vi "EditorThumbnail addNewData.vi"(7 "limit":T1={"plotIdx"=-1, "Minimum"=-inf, "Maximum"=inf}, 8 "error in (no error)":errorcluster, 11 "EditorThumbnail in":refnum<class "EditorThumbnail.lvclass">) -> (0 "error out":errorcluster, 3 "EditorThumbnail out":refnum<class "EditorThumbnail.lvclass">)   [LabVIEW 2018, in "EditorThumbnail.lvclass"]
uses:
  EditorThumbnail.lvclass
  EditorThumbnail.lvclass/EditorThumbnail.ctl
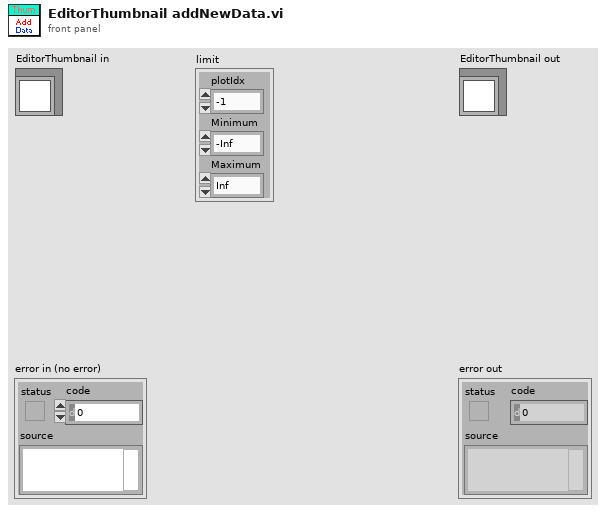
[diagram p1: front panel]
types:
  T1 = cluster{"plotIdx":i32, "Minimum":dbl, "Maximum":dbl}
  T2 = cluster{"index":u32, "data":cluster{"xdata":dbl[], "ydata":sgl[]}[], "peak":dbl[], "picture":picture}[]
  T3 = cluster{"index":u32, "data":cluster{"xdata":dbl[], "ydata":sgl[]}[], "peak":dbl[], "picture":picture}
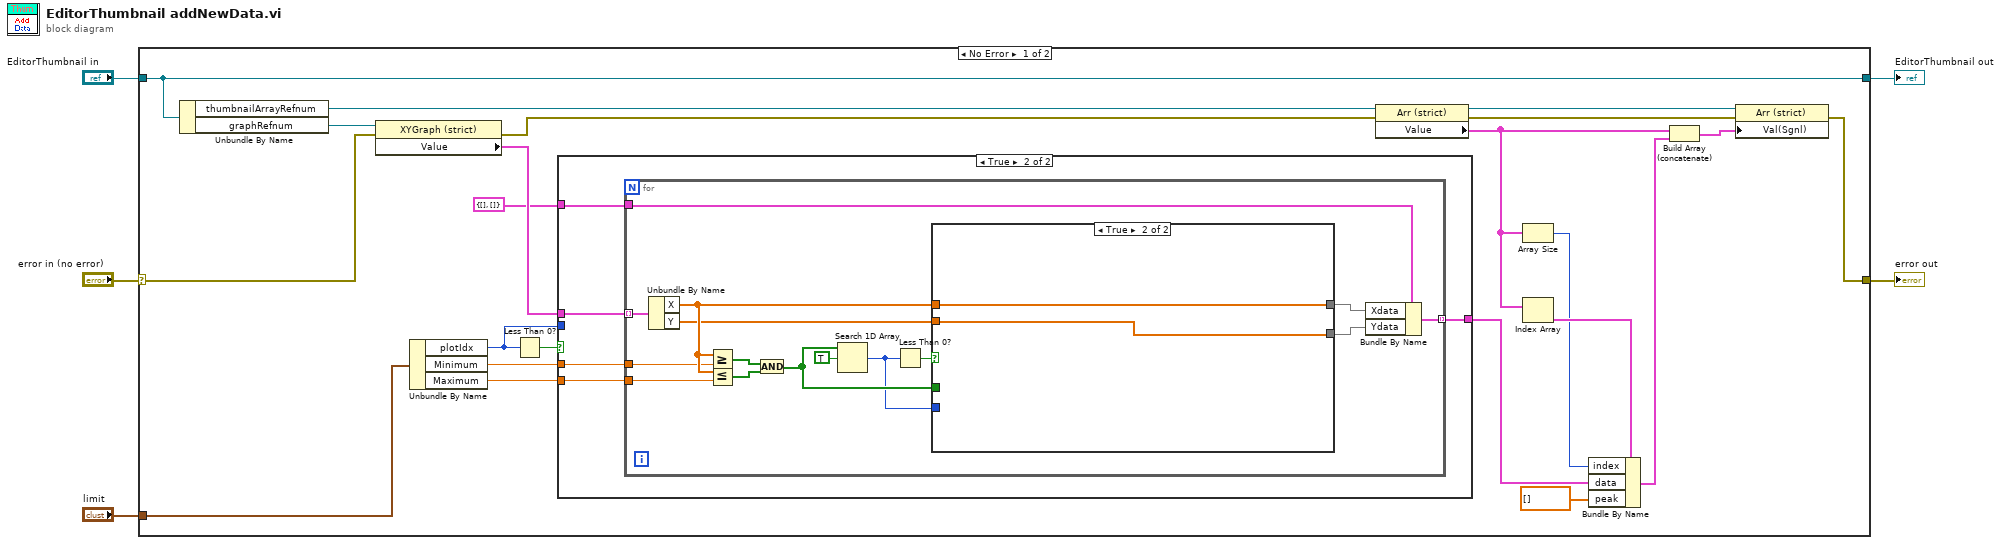
[diagram p0: block diagram]
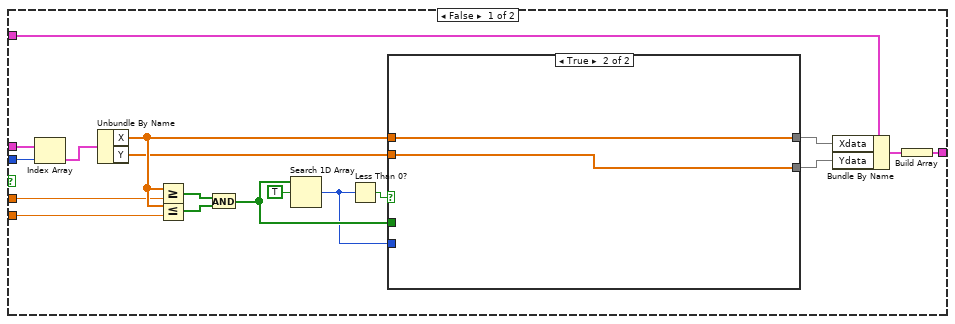
[diagram p2: hidden frame]
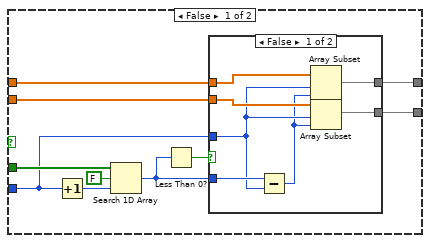
[diagram p3: hidden frame]
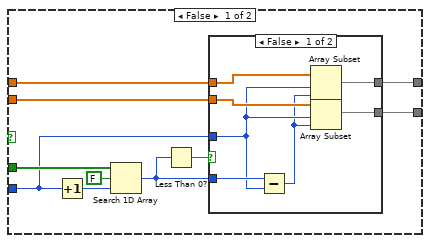
[diagram p5: hidden frame]
diagram:
  n1 = case shown="No Error" "error in (no error)" {
    selector: "error in (no error)" -> [w7 w109]
    tunnel: [w6 w109] -> w4
    tunnel: [w21 w108] -> w2
    tunnel: "EditorThumbnail in" -> [w21 w108]
    tunnel: "limit" -> [w16 _]
    frame No Error {
      n2 = Unbundle By Name(w21) -> ("thumbnailArrayRefnum"=w20:refnum<vi>, "graphRefnum"=w14:refnum<vi>)
      n3 = property class="XYGraph (strict)"(reference=w14, error in=w7) -> (error out=w13:errorcluster, "Value"=w12:cluster{"X":dbl[], "Y":sgl[]}[])  [unwired: 1 out]
      n4 = Unbundle By Name(w16) -> ("plotIdx"=w9:i32, "Minimum"=w11:dbl, "Maximum"=w10:dbl)
      n5 = Less Than 0?(x=w9) -> (x < 0?=w15:bool)
      n6 = case shown="True" w15 {
        tunnel: [w28 w71] -> w19
        tunnel: w12 -> [w45 w70]
        tunnel: w11 -> [w33 w69]
        tunnel: w10 -> [w31 w68]
        tunnel: w9 -> [w44 _]
        tunnel: cluster{"Xdata":dbl[], "Ydata":sgl[]} {"Xdata"=[], "Ydata"=[]} -> [w30 w67]
        frame False {
          n7 = Index Array(array=w45, index=w44) -> (element=w32:cluster{"X":dbl[], "Y":sgl[]})
          n8 = Unbundle By Name(w32) -> ("X"=w35:dbl[], "Y"=w34:sgl[])
          n9 = Greater Or Equal?(x=w35, y=w33) -> (x >= y?=w43:bool[])
          n10 = Less Or Equal?(x=w35, y=w31) -> (x <= y?=w42:bool[])
          n11 = And(x=w43, y=w42) -> (x .and. y?=w39:bool[])
          n12 = Search 1D Array(1D array=w39, element=TRUE) -> (index of element=w38:i32)  [unwired: 1 in]
          n13 = Less Than 0?(x=w38) -> (x < 0?=w40:bool)
          n14 = case shown="True" w40 {
            tunnel: w39 -> [w54 _]
            tunnel: w38 -> [w50 _]
            tunnel: w35 -> [w49 w66]
            tunnel: w34 -> [w46 w65]
            tunnel: [w48 w66] -> w37
            tunnel: [w47 w65] -> w36
            frame False {
              n15 = Increment(x=w50) -> (x+1=w55:i32)
              n16 = Search 1D Array(1D array=w54, element=FALSE, start index (0)=w55) -> (index of element=w51:i32)
              n17 = Less Than 0?(x=w51) -> (x < 0?=w52:bool)
              n18 = case shown="False" w52 {
                tunnel: w51 -> [w58 _]
                tunnel: w50 -> [w57 _]
                tunnel: w49 -> [w62 w64]
                tunnel: [w60 w64] -> w48
                tunnel: [w59 w63] -> w47
                tunnel: w46 -> [w61 w63]
                frame False {
                  n19 = Subtract(x=w58, y=w57) -> (x-y=w56:i32)
                  n20 = Array Subset(array=w62, index=w57, length=w56) -> (w60:dbl[])
                  n21 = Array Subset(array=w61, index=w57, length=w56) -> (w59:sgl[])
                }
                frame True {
                }
              }
            }
            frame True {
            }
          }
          n22 = Bundle By Name(cluster=w30, "Xdata"=w37, "Ydata"=w36) -> (w29:cluster{"Xdata":dbl[], "Ydata":sgl[]})
          n23 = Build Array(w29) -> (w28:cluster{"Xdata":dbl[], "Ydata":sgl[]}[])
        }
        frame True {
          n24 = for {
            tunnel: w70 -> [w77] mode=indexing
            tunnel: [w86] -> w71 mode=indexing
            tunnel: w69 -> [w74]
            tunnel: w68 -> [w73]
            tunnel: w67 -> [w72]
            n25 = Unbundle By Name(w77) -> ("X"=w76:dbl[], "Y"=w75:sgl[])
            n26 = Greater Or Equal?(x=w76, y=w74) -> (x >= y?=w85:bool[])
            n27 = Less Or Equal?(x=w76, y=w73) -> (x <= y?=w84:bool[])
            n28 = And(x=w85, y=w84) -> (x .and. y?=w81:bool[])
            n29 = Search 1D Array(1D array=w81, element=TRUE) -> (index of element=w80:i32)  [unwired: 1 in]
            n30 = Less Than 0?(x=w80) -> (x < 0?=w82:bool)
            n31 = case shown="True" w82 {
              tunnel: w81 -> [w95 _]
              tunnel: w80 -> [w91 _]
              tunnel: w76 -> [w90 w107]
              tunnel: w75 -> [w87 w106]
              tunnel: [w89 w107] -> w79
              tunnel: [w88 w106] -> w78
              frame False {
                n32 = Increment(x=w91) -> (x+1=w96:i32)
                n33 = Search 1D Array(1D array=w95, element=FALSE, start index (0)=w96) -> (index of element=w92:i32)
                n34 = Less Than 0?(x=w92) -> (x < 0?=w93:bool)
                n35 = case shown="False" w93 {
                  tunnel: w92 -> [w99 _]
                  tunnel: w91 -> [w98 _]
                  tunnel: w90 -> [w103 w105]
                  tunnel: [w101 w105] -> w89
                  tunnel: [w100 w104] -> w88
                  tunnel: w87 -> [w102 w104]
                  frame False {
                    n36 = Subtract(x=w99, y=w98) -> (x-y=w97:i32)
                    n37 = Array Subset(array=w103, index=w98, length=w97) -> (w101:dbl[])
                    n38 = Array Subset(array=w102, index=w98, length=w97) -> (w100:sgl[])
                  }
                  frame True {
                  }
                }
              }
              frame True {
              }
            }
            n39 = Bundle By Name(cluster=w72, "Xdata"=w79, "Ydata"=w78) -> (w86:cluster{"Xdata":dbl[], "Ydata":sgl[]})
          }
        }
      }
      n40 = property class="Arr (strict)"(reference=w20, error in=w13) -> (reference out=w18:refnum<vi>, error out=w17:errorcluster, "Value"=w27:T2)
      n41 = Array Size(array=w27) -> (size(s)=w25:i32)
      n42 = Index Array(array=w27) -> (element=w26:T3)  [unwired: 1 in]
      n43 = Bundle By Name(cluster=w26, "index"=w25, "data"=w19, "peak"=dbl[] []) -> (w24:T3)
      n44 = Build Array (concatenate)(w27, w24) -> (w23:T2)
      n45 = property class="Arr (strict)"(reference=w18, error in=w17, "Val(Sgnl)"=w23) -> (error out=w6:errorcluster)  [unwired: 1 out]
    }
    frame Error {
    }
  }
  "error out" <- w4
  "EditorThumbnail out" <- w2
